vi "SEA_position_PI_testing.vi"() -> ()   [LabVIEW 2019]
uses:
  <vilib>/FPGAPlugInAG/sbRIO-9627/niLvFpga_Open_sbRIO-9627.vi
  <vilib>/rvi/interface/common/dynamic/niFpgaDynamicAddResources.vi
  <vilib>/Utility/error.llb/Error Cluster From Error Code.vi
  <vilib>/rvi/errors/niLvFpgaAdjustHostInterfaceError.vi
  <vilib>/addons/control/pid/pid.llb/PID (DBL).vi
  <vilib>/FPGAPlugInAG/Dynamic/niLvFpga_Close_Dynamic.vi
  <vilib>/rvi/interface/nirviOpenFPGA/nirviOpenFPGA.xnode
  FPGA Bitfiles/ccmultiplier_FPGATarget_CCPItesting_ybhjPyRilUw.lvbitx
  CC_PI_testing.vi
  <vilib>/rvi/interface/nirviReadWriteControl/nirviReadWriteControl.xnode
  <vilib>/rvi/interface/nirviCloseFPGA/nirviCloseFPGA.xnode
  <vilib>/addons/control/pid/NI_PID_pid.lvlib
  NiFpgaLv.dll
  <vilib>/rvi/interface/Simulation/niFpgaSimulationCallBeginRW.vi
panel:
  out "Current":dynamicdata(graph)
  out "Position":dynamicdata(graph)
  in  "Position PID gains":T1={"proportional gain (Kc)"=1.0, "integral time (Ti, min)"=0.01, "derivative time (Td, min)"=0.0} {"derivative time (Td, min)" format="%.3f"; "integral time (Ti, min)" format="%.3f"; "proportional gain (Kc)" format="%.3f"}
  in  "amplitude":sgl
  in  "Fre":sgl
  out "dutycycle":sgl(graph)
  out "raw current":sgl
  out "motor direction":bool
  out "filtered motor position radians":sgl(graph)
  out "error %":sgl(knob) scale=-100.0..100.0
  in  "weighting term encoder joint":sgl
  in  "weighting term encoder motor":sgl
  in  "Position Reset motor side":bool
  in  "Position Reset joint side":bool
  in  "Ki":sgl
  in  "Kp":sgl
  in  "zero Value M2":sgl
  in  "weighting term(M2)":sgl
  in  "stop":bool
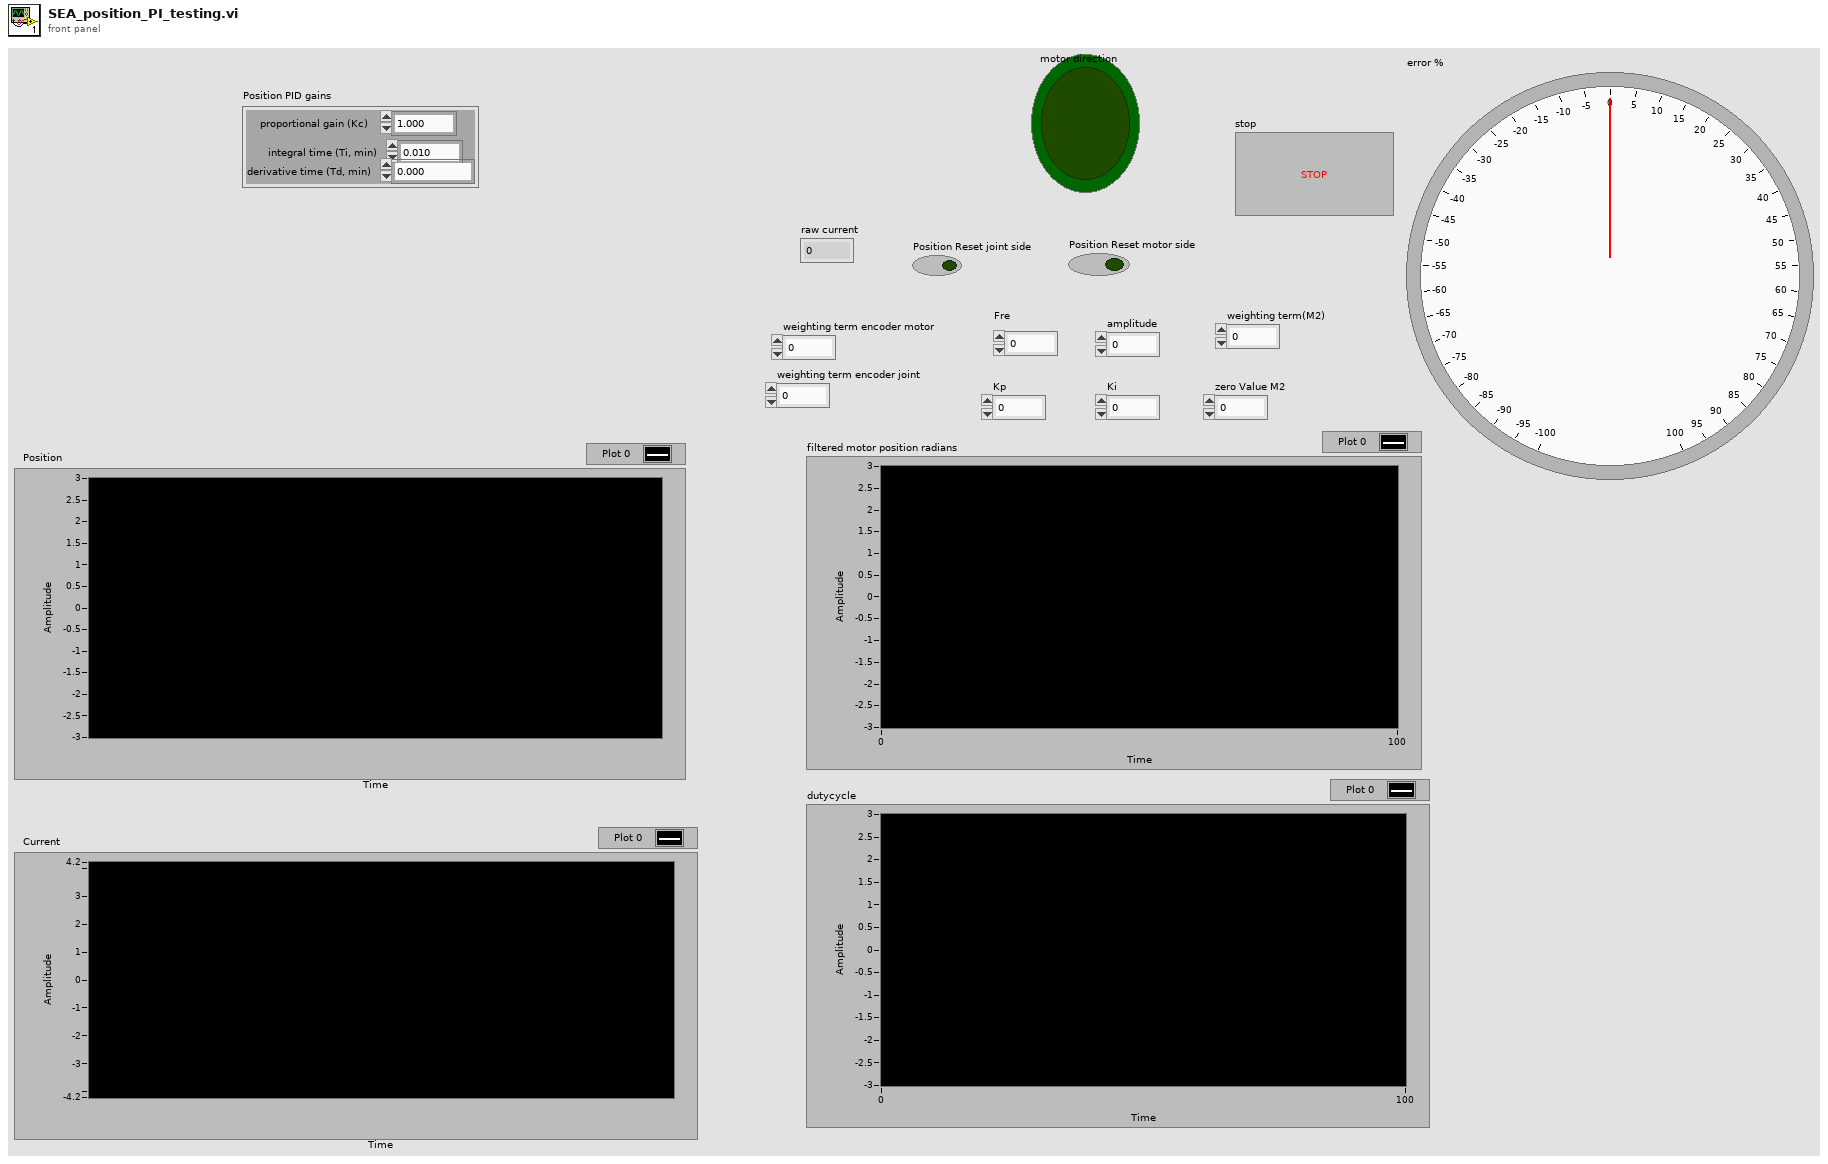
[diagram p1: front panel]
types:
  T1 = cluster{"proportional gain (Kc)":dbl, "integral time (Ti, min)":dbl, "derivative time (Td, min)":dbl}
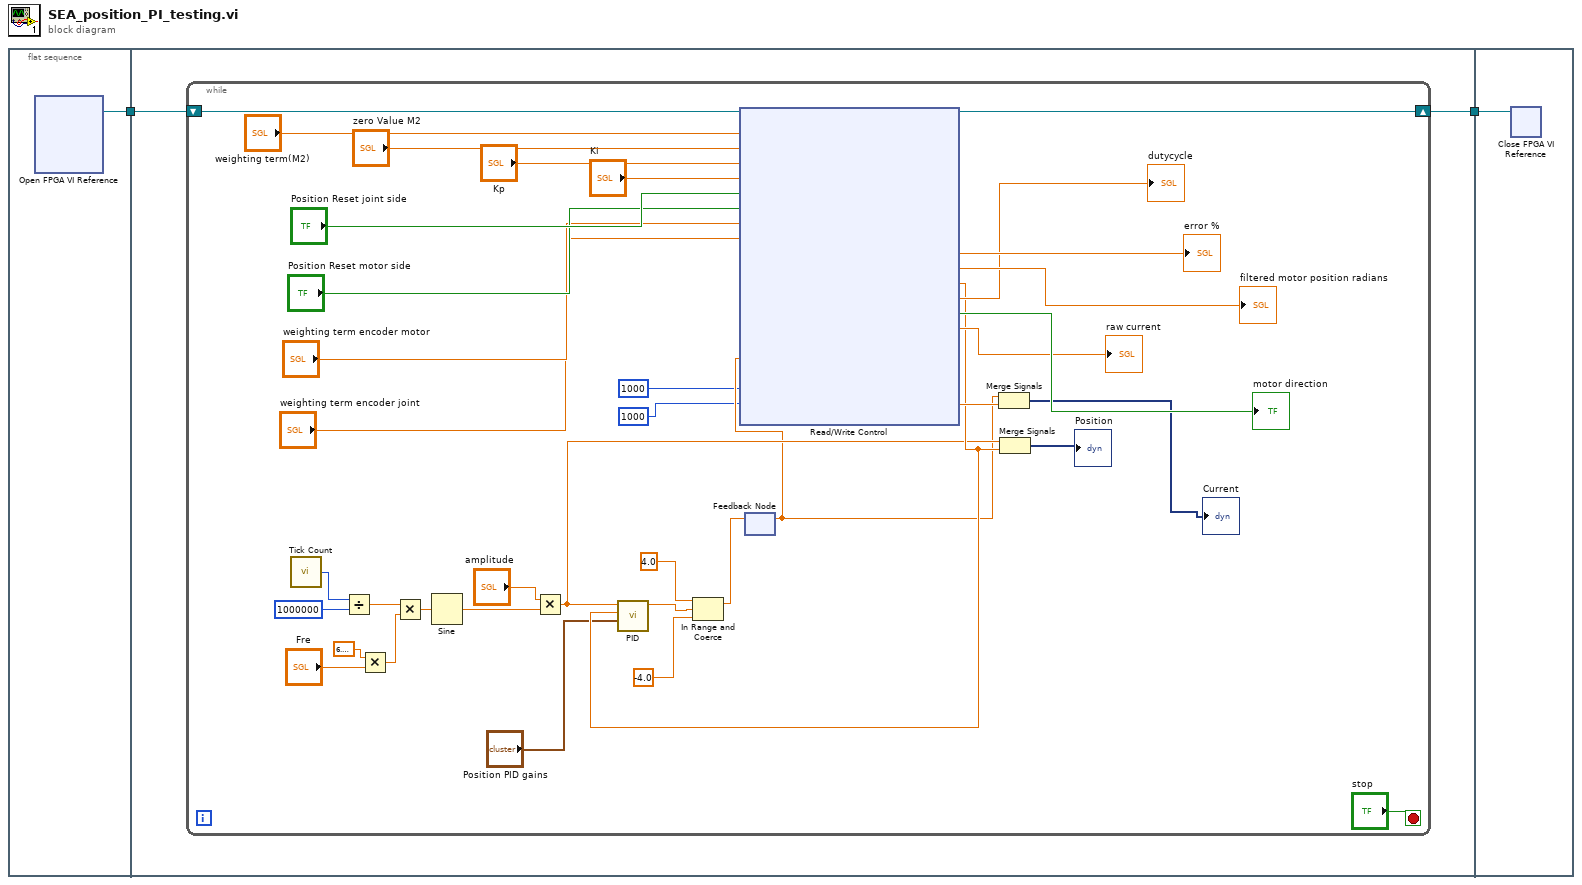
[diagram p0: block diagram]
diagram:
  n1 = flat-sequence {
    tunnel: [w3] -> w2
    tunnel: w2 -> [w5]
    tunnel: [w4] -> w1
    tunnel: w1 -> [w44]
    frame #0 {
      n2 = xnode "Open FPGA VI Reference"() -> ("FPGA VI Reference Out"=w3:refnum<k20>)  [unwired: 2 in, 1 out]
    }
    frame #1 {
      n3 = while {
        shift-right: [w42] -> w4
        shift-left: w5 -> [w43]
        stop <- "stop" stop-if-true
        n4 = call "Tick Count"() -> ("Tick Count(uSec)"=w20:u32)
        n5 = Divide(x=w20, y=u32 1000000) -> (x/y=w26:dbl)
        n6 = Multiply(x=sgl 6.2831855, y="Fre") -> (x*y=w21:sgl)
        n7 = Multiply(x=w26, y=w21) -> (x*y=w22:dbl)
        n8 = Sine(x=w22) -> (sin(x)=w25:dbl)
        n9 = Multiply(x="amplitude", y=w25) -> (x*y=w11:dbl)
        n10 = feedback #1() -> (w10:dbl)  [unwired: 1 in]
        n11 = xnode "Read/Write Control"("FPGA VI Reference In"=w43, "weighting term(M2)"="weighting term(M2)", "zero Value M2"="zero Value M2", "Kp"="Kp", "Ki"="Ki", "Position Reset joint side"="Position Reset joint side", "Position Reset motor side"="Position Reset motor side", "weighting term encoder motor"="weighting term encoder motor", "weighting term encoder joint"="weighting term encoder joint", "reference"=w10, "Velocity Interval (uSec)  joint side"=i16 1000, "Velocity Interval (uSec)  motor side"=i16 1000) -> ("FPGA VI Reference Out"=w42:refnum<k20>, "error %"=→"error %":sgl, "filtered motor position radians"=→"filtered motor position radians":sgl, "filtered joint position radians"=w17:sgl, "control_ip"=→"dutycycle":sgl, "motor direction"=→"motor direction":bool, "raw current"=→"raw current":sgl, "Filtered Current(M2)"=w28:sgl)  [unwired: 1 in, 3 out]
        n12 = call-poly <vilib>:"PID.vi"("PID gains"="Position PID gains", "process variable"=w17, "setpoint"=w11) -> ("output"=w15:dbl)  [unwired: 7 in, 1 out]
        n13 = In Range and Coerce(upper limit=4.0, x=w15, lower limit=-4.0) -> (coerced(x)=w12:dbl)  [unwired: 1 out]
        n14 = feedback-in #1(w12) -> ()
        n15 = Merge Signals(w10, w28) -> (→"Current":dynamicdata)
        n16 = Merge Signals(w11, w17) -> (→"Position":dynamicdata)
      }
    }
    frame #2 {
      n17 = xnode "Close FPGA VI Reference"("FPGA VI Reference In"=w44) -> ()  [unwired: 1 in, 1 out]
    }
  }
